vi "SearchDatabase.vi"(0 "Licence":string, 1 "Image in":T1, 2 "Database":string[][](array[string]), 5 "error in":errorcluster) -> (6 "Individual":T2, 8 "error out":errorcluster)   [LabVIEW 2019]
uses:
  <vilib>/vision/Image Controls.llb/IMAQ Image.ctl
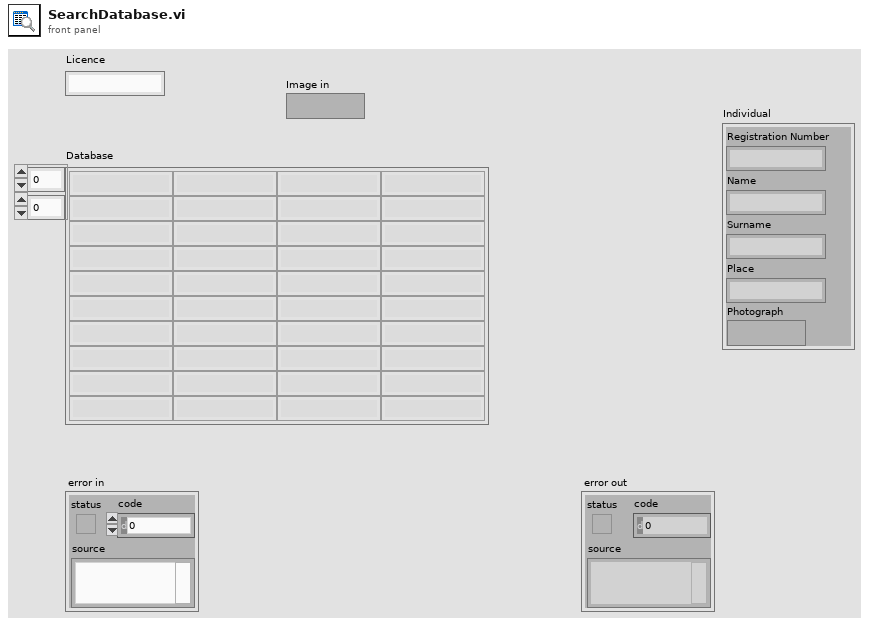
[diagram p1: front panel]
types:
  T1 = typedef "IMAQ Image.ctl" = refnum<image>
  T2 = cluster{"Registration Number":string, "Name":string, "Surname":string, "Place":string, "Photograph":T1}
  T3 = cluster{"Registration Number":string, "Name":string, "Surname":string, "Vehicle":string, "Photograph":T1}
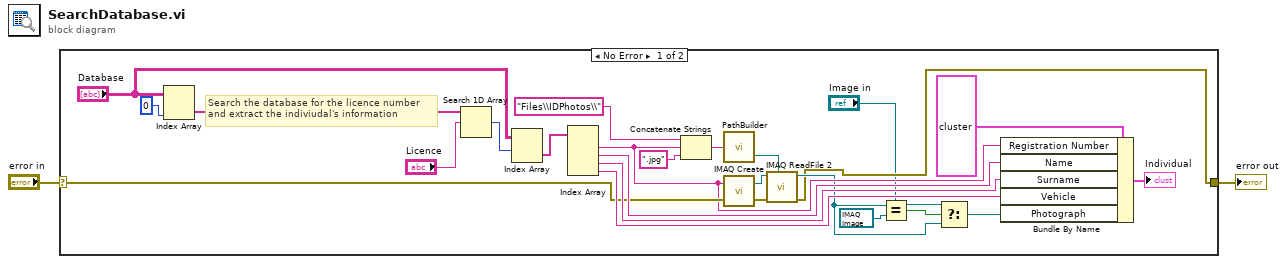
[diagram p0: block diagram]
diagram:
  n1 = case shown="No Error" "error in" {
    selector: "error in" -> [w11 w28]
    tunnel: [w4 w28] -> w1
    frame No Error {
      # "Search the database for the licence number\nand extract the indiviudal's information"
      n2 = Index Array(array="Database", index (col)=0 ("disabled index (col)")) -> (element=w27:string[])  [unwired: 1 in]
      n3 = Search 1D Array(1D array=w27, element="Licence") -> (index of element=w23:i32)  [unwired: 1 in]
      n4 = Index Array(array="Database", index (row)=w23) -> (element=w21:string[])  [unwired: 1 in]
      n5 = Index Array(array=w21) -> (element #1=w9:string, element #2=w20:string, element #3=w19:string, element #4=w18:string)  [unwired: 4 in]
      n6 = Concatenate Strings("Files\\IDPhotos\\" ("string"), w9, ".jpg" ("string")) -> (w15:string)
      n7 = call "PathBuilder.vi"("Path (String)"=w15) -> ("Path (Path)"=w14:path)  [unwired: 1 out]
      n8 = call "IMAQ Create"("Image Name"=w9, "error in (no error)"=w11) -> ("New Image"=w12:T1, "error out"=w10:errorcluster)  [unwired: 3 in]
      n9 = call "IMAQ ReadFile 2"("File Path"=w14, "error in (no error)"=w10, "Image"=w12) -> ("error out"=w4:errorcluster, "Image Out"=w5:T1)  [unwired: 4 in, 3 out]
      n10 = Equal?(x=w5, y=T1 refnum ("Photograph")) -> (x = y?=w7:bool)
      n11 = Select(t="Image in", s=w7, f=w5) -> (s? t:f=w6:T1)
      n12 = Bundle By Name(cluster=T3 {"Registration Number"="", "Name"="", "Surname"="", "Vehicle"="", "Photograph"=refnum} ("IndividualCluster"), "Registration Number"=w9, "Name"=w20, "Surname"=w19, "Vehicle"=w18, "Photograph"=w6) -> (→"Individual":T3)
    }
    frame Error {
    }
  }
  "error out" <- w1
